vi "BigIntIsPrime.vi"(1 "a":cluster{"Boolean":bool, "Array":u64[]}) -> (0 "Is Prime":bool)   [LabVIEW 2023]
panel:
  # "s"
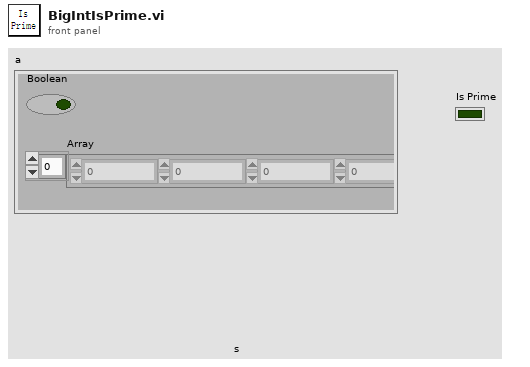
[diagram p1: front panel]
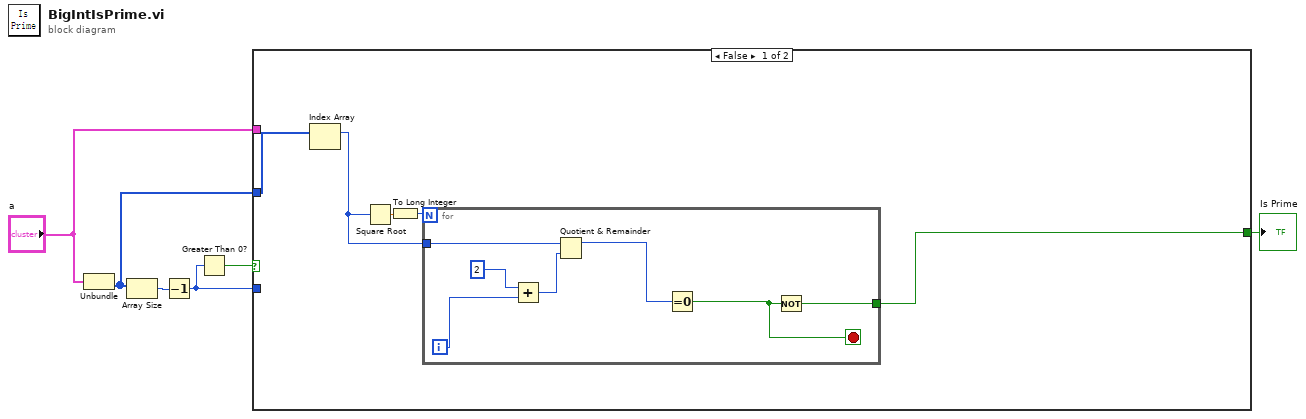
[diagram p0: block diagram]
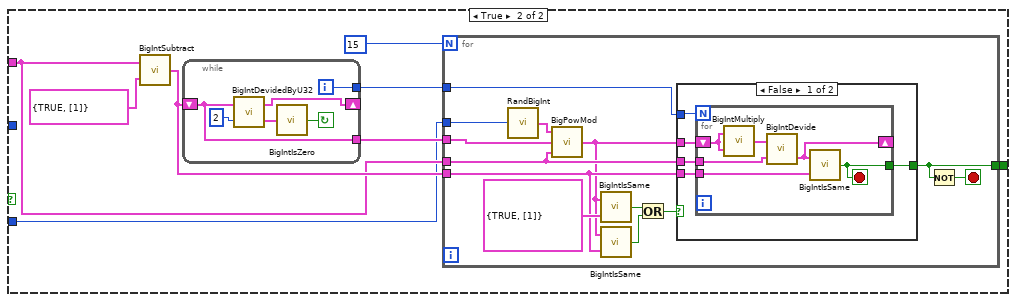
[diagram p2: hidden frame]
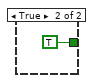
[diagram p3: hidden frame]
diagram:
  n1 = Unbundle("a") -> ("Array"=w1:u64[])  [unwired: 1 out]
  n2 = Array Size(array=w1) -> (size(s)=w5:i32)
  n3 = Decrement(x=w5) -> (x-1=w3:i32)
  n4 = Greater Than 0?(x=w3) -> (x > 0?=w2:bool)
  n5 = case shown="False" w2 {
    tunnel: [w7 w21] -> w6
    tunnel: "a" -> [_ w20]
    tunnel: w3 -> [_ w19]
    tunnel: w1 -> [w11 _]
    frame False {
      n6 = Index Array(array=w11) -> (element=w10:u64)  [unwired: 1 in]
      n7 = Square Root(x=w10) -> (sqrt(x)=w8:dbl)
      n8 = To Long Integer(number=w8) -> (32bit integer=w9:i32)
      n9 = for {
        N: w9 -> [_]
        tunnel: w10 -> [w18]
        tunnel: [w13] -> w7
        i -> [w17]
        stop <- w12 stop-if-true
        n10 = Add(x=2, y=w17) -> (x+y=w15:i32)
        n11 = Quotient & Remainder(x=w18, y=w15) -> (x-y*floor(x/y)=w14:u64)  [unwired: 1 out]
        n12 = Equal To 0?(x=w14) -> (x = 0?=w12:bool)
        n13 = Not(x=w12) -> (.not. x?=w13:bool)
      }
    }
    frame True {
      n14 = call "BigIntSubtract.vi"("b"=cluster{bool, u64[]} {TRUE, [1]}, "a"=w20) -> ("a - b"=w23:cluster{"Boolean":bool, "Array":u64[]})
      n15 = while {
        shift-right: [w55] -> _
        shift-left: w23 -> [w52]
        tunnel: [w54] -> w22
        tunnel: [w52] -> w24
        i -> [w54]
        stop <- w56 continue-if-true
        n16 = call "BigIntDevidedByU32.vi"("b (<1e9)"=u64 2, "a"=w52) -> ("a % b"=w53:cluster{"Boolean":bool, "Array":u64[]}, "a / b"=w55:cluster{"Boolean":bool, "Array":u64[]})
        n17 = call "BigIntIsZero.vi"("a"=w53) -> ("a = 0"=w56:bool)
      }
      n18 = for {
        N: 15 -> [_]
        tunnel: w24 -> [w39]
        tunnel: w20 -> [w32]
        tunnel: w23 -> [w31]
        tunnel: w22 -> [w33]
        tunnel: [w30] -> w21
        tunnel: w19 -> [w27]
        stop <- w34 stop-if-true
        n19 = call "RandBigInt.vi"("length (x1e9)"=w27) -> ("Random Number"=w29:cluster{"P/N":bool, "Array":u64[]})
        n20 = call "BigPowMod.vi"("c"=w32, "b"=w39, "a"=w29) -> ("a ^ b mod c"=w28:cluster{"Boolean":bool, "Array":u64[]})
        n21 = call "BigIntIsSame.vi"("b"=cluster{bool, u64[]} {TRUE, [1]}, "a"=w28) -> ("a = b"=w36:bool)
        n22 = call "BigIntIsSame.vi"("b"=w31, "a"=w28) -> ("a = b"=w35:bool)
        n23 = Or(x=w36, y=w35) -> (x .or. y?=w37:bool)
        n24 = case shown="False" w37 {
          tunnel: w33 -> [w44 _]
          tunnel: w28 -> [w43 _]
          tunnel: w32 -> [w42 _]
          tunnel: w31 -> [w41 _]
          tunnel: [w40 TRUE] -> w30
          frame False {
            n25 = for {
              N: w44 -> [_]
              shift-right: [w46] -> _
              shift-left: w43 -> [w50]
              tunnel: w42 -> [w48]
              tunnel: w41 -> [w47]
              tunnel: [w45] -> w40
              stop <- w45 stop-if-true
              n26 = call "BigIntMultiply.vi"("b"=w50, "a"=w50) -> ("a * b"=w49:cluster{"Boolean":bool, "Array":u64[]})
              n27 = call "BigIntDevide.vi"("b"=w48, "a"=w49) -> ("a % b"=w46:cluster{"Boolean":bool, "Array":u64[]})  [unwired: 1 out]
              n28 = call "BigIntIsSame.vi"("b"=w47, "a"=w46) -> ("a = b"=w45:bool)
            }
          }
          frame True {
          }
        }
        n29 = Not(x=w30) -> (.not. x?=w34:bool)
      }
    }
  }
  "Is Prime" <- w6
